vi "Handle Exception.vi"(7 "Inputs":T2, 8 "error in (no error)":errorcluster, 11 "FileNotFoundException in":refnum<class "FileNotFoundException.lvclass">) -> (0 "error out":errorcluster, 5 "Outputs":T1)   [LabVIEW 2020, in "HTTP Server.lvlib" / "FileNotFoundException.lvclass"]
uses:
  FileNotFoundException.lvclass
  Exception Inputs.ctl
  Values/Values.lvclass
  <vilib>/IlluminatedG/IG HTTP Utils/HTTP Utils/Request/Request.lvclass
  <vilib>/IlluminatedG/IG HTTP Utils/HTTP Utils/Response/Response.lvclass
  <vilib>/IlluminatedG/lv-stream/URI/URI.lvclass
  Session/Session.lvclass
  Exception Outputs.ctl
  File Response/File Response.lvclass
  FileNotFoundException.lvclass/FileNotFoundException.ctl
  <vilib>/Utility/error.llb/DialogType.ctl
  HTTP Server.lvlib
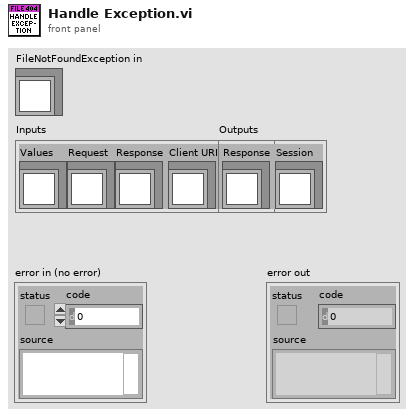
[diagram p1: front panel]
types:
  T1 = typedef "HTTP Server.lvlib/Exception Outputs.ctl" = cluster{"Response":refnum<class "Response.lvclass">, "Session":refnum<class "Session.lvclass">}
  T2 = typedef "HTTP Server.lvlib/Exception Inputs.ctl" = cluster{"Values":refnum<class "Values.lvclass">, "Request":refnum<class "Request.lvclass">, "Response":refnum<class "Response.lvclass">, "Client URI":refnum<class "URI.lvclass">, "Session":refnum<class "Session.lvclass">}
  T3 = typedef "DialogType.ctl" = u16
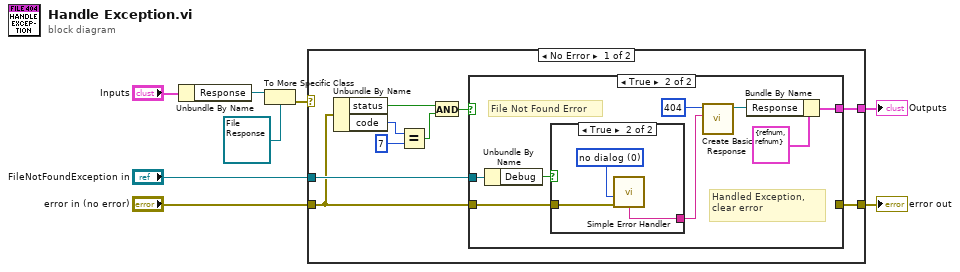
[diagram p0: block diagram]
diagram:
  n1 = Unbundle By Name("Inputs") -> ("Response"=w1:refnum<class "Response.lvclass">)
  n2 = To More Specific Class(target class=refnum<class "File Response.lvclass"> refnum ("HTTP Server.lvlib:File Response.lvclass"), reference=w1) -> (error out=w7:errorcluster)  [unwired: 1 in, 1 out]
  n3 = case shown="No Error" w7 {
    tunnel: "FileNotFoundException in" -> [w12 _]
    tunnel: "error in (no error)" -> [w9 w30]
    tunnel: [w11 w30] -> w4
    tunnel: [w10 _] -> w3
    frame No Error {
      n4 = Unbundle By Name(w9) -> ("status"=w15:bool, "code"=w17:i32)
      n5 = Equal?(x=w17, y=7) -> (x = y?=w14:bool)
      n6 = And(x=w15, y=w14) -> (x .and. y?=w13:bool)
      n7 = case shown="True" w13 {
        tunnel: w12 -> [_ w24]
        tunnel: w9 -> [w18 w22]
        tunnel: [w18 _] -> w11
        tunnel: [_ w19] -> w10
        frame False {
          # "Not a File Not Found Error"
        }
        frame True {
          # "Handled Exception, clear error"
          # "File Not Found Error"
          n8 = Unbundle By Name(w24) -> ("Debug"=w23:bool)
          n9 = case shown="True" w23 {
            tunnel: [_ w27] -> w25
            tunnel: w22 -> [_ w29]
            frame False {
            }
            frame True {
              w28 = T3 0 items=["no dialog", "OK message", "continue or stop message", "OK message + warnings", "continue/stop + warnings"] ("type of dialog (OK msg:1)")
              n10 = call <vilib>:"Simple Error Handler.vi"("type of dialog (OK msg:1)"=w28, "error in (no error)"=w29) -> ("message"=w27:string)  [unwired: 3 in, 4 out]
            }
          }
          n11 = call <vilib>:"Create Basic Response.vi"("Payload"=w25, "Status Code"=u16 404 ("Status Code (200)")) -> ("Response out"=w20:refnum<class "Response.lvclass">)  [unwired: 8 in, 1 out]
          n12 = Bundle By Name(cluster=T1 {"Response"=refnum, "Session"=refnum} ("Outputs"), "Response"=w20) -> (w19:T1)
        }
      }
    }
    frame Error {
      # "Not a FileResponse instance"
      # "Not a FileResponse, don't care about it."
    }
  }
  "error out" <- w4
  "Outputs" <- w3
